vi "Convert I2C Transaction.vi"(8 "error in (no error)":errorcluster, 11 "I2C Transaction":string[][](array[string])) -> (0 "error out":errorcluster, 3 "U8 Array":u8[](array[numeric]))   [LabVIEW 2025, in "I2C Bus Monitor.lvclass"]
uses:
  I2C Bus Monitor.lvclass
  I2C Bus Monitor.lvclass/I2C Bus Monitor.ctl
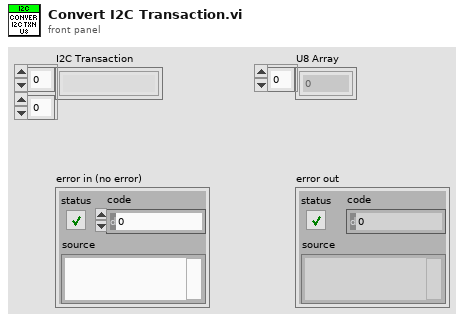
[diagram p1: front panel]
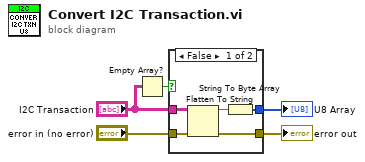
[diagram p0: block diagram]
diagram:
  n1 = Empty Array?(array="I2C Transaction") -> (empty?=w2:bool)
  n2 = case shown="False" w2 {
    tunnel: "error in (no error)" -> [w10 w11]
    tunnel: [w9 w11] -> w4
    tunnel: [w6 _] -> w3
    tunnel: "I2C Transaction" -> [w8 _]
    frame False {
      n3 = Flatten To String(anything=w8, error in (no error)=w10) -> (data string=w7:string, error out=w9:errorcluster)  [unwired: 2 in, 1 out]
      n4 = String To Byte Array(string=w7) -> (unsigned byte array=w6:u8[])
    }
    frame True {
    }
  }
  "error out" <- w4
  "U8 Array" <- w3
